vi "LightSheetController_Main.vi"() -> ()   [LabVIEW 2018]
uses:
  VISource/SubVI/ConfigParameters_Analog.ctl
  VISource/SubVI/ConfigParameters_Others1.ctl
  VISource/SubVI/ConfigParameters_Others2.ctl
  VISource/SubVI/ConfigParameters_Digital.ctl
  VISource/SubVI/SetupInfo.ctl
  VISource/SubVI/ProcessParametersOut.ctl
  VISource/SubVI/WaveformParameters.ctl
  VISource/SubVI/AnalogWaveform.ctl
  VISource/SubVI/DigitalWaveform.ctl
  VISource/SubVI/PhysicalResource.ctl
  VISource/SubVI/ControlsRef.ctl
panel:
  in  "FunctionSelect":enum32{"Control Panel", "Settings", "About"}(tab)=enum."Settings"
  in  "XYOnlyMode":bool
  out "RunningMode":string caption="Running Mode"
  in  "QuitRunning":bool
  in  "EXIT":bool
  in  "Mode_1":bool
  in  "Mode_2A":bool
  in  "Mode_2B":bool
  out "ElapsedTime":dbl caption="Elapsed Time" format="%.2f sec"
  in  "EventDetectionMode":bool
  in  "StimulationMode":bool
  out "Messages":string
  in  "ConfigParameters_Digital":T1={"Steps per volume"=25.0, "Time per volume (s)"=0.4, "OG start layer"=23.0, "Objective Lin Rising Vel (micron/ms）"=1.0, "Image depth (micron)"=200.0, "OG latency (s)"=10.0, "OG repitation"=3.0, "OG end layer"=25.0, "Shock1 duration (s)"=0.001, "Shock2 duration (s)"=0.001, "Shock3 duration (s)"=0.01, "Shock4 duration (s)"=0.01, "Shock5 duration (s)"=0.1, "Shock duration_New"=[0.001, 0.001, 0.01, 0.01, 0.1]}
  in  "ConfigParameters_Analog":T2={"JAI camera fps"=100.0, "Bi-Lateral Galvo xy scan range (V)"=0.6, "Bi-Lateral Galvo xy scan frequency (Hz)"=500, "AOM Blind percent (%)"=0.1, "AOM start blind percent (%) "=70.0, "ROI threshold"=3.0, "AO Sampling rate"=500000.0} {"AOM start blind percent (%)" min=10.0 max=90.0; "AOM Blind percent (%)" min=0.1 max=100.0; "Bi-Lateral Galvo xy scan frequency (Hz)" min=500 max=500; "Bi-Lateral Galvo xy scan range (V)" min=0.0 max=1.5}
  in  "ConfigParameters_Other1":T3={"Frontal Galvo xy scan range (V)"=0.14, "Frontal Galvo xy scan frequency (Hz)"=500, "PFI 0 digital clock frequency"=500000.0, "Window size for layer index"=0.5, "sCMOS fps"=95.0} {"Frontal Galvo xy scan frequency (Hz)" min=500 max=500; "Frontal Galvo xy scan range (V)" min=0.0 max=1.5}
  in  "ConfigParameters_Others2":T4={"#Trials baseline"=6, "#Trials test"=6, "Time before acq. (s)"=360.0, "Time before test (s)"=600.0, "#Blocks acquisition"=5, "Inter-trial interval baseline (s)"=60.0, "#Trials per acquition block"=6, "Inter-block interval acquisition (s)"=360.0, "Inter-trial interval acquisition (s)"=20.0, "Flash latency (s)"=20.0, "Flash duration (s)"=3.2, "Response duration (s)"=40.0, "MaxTimeEventDetection (s)"=3600, "StimType"=enum."Flash", "#MaxEvents"=10}
  # "Light Sheet Controller"
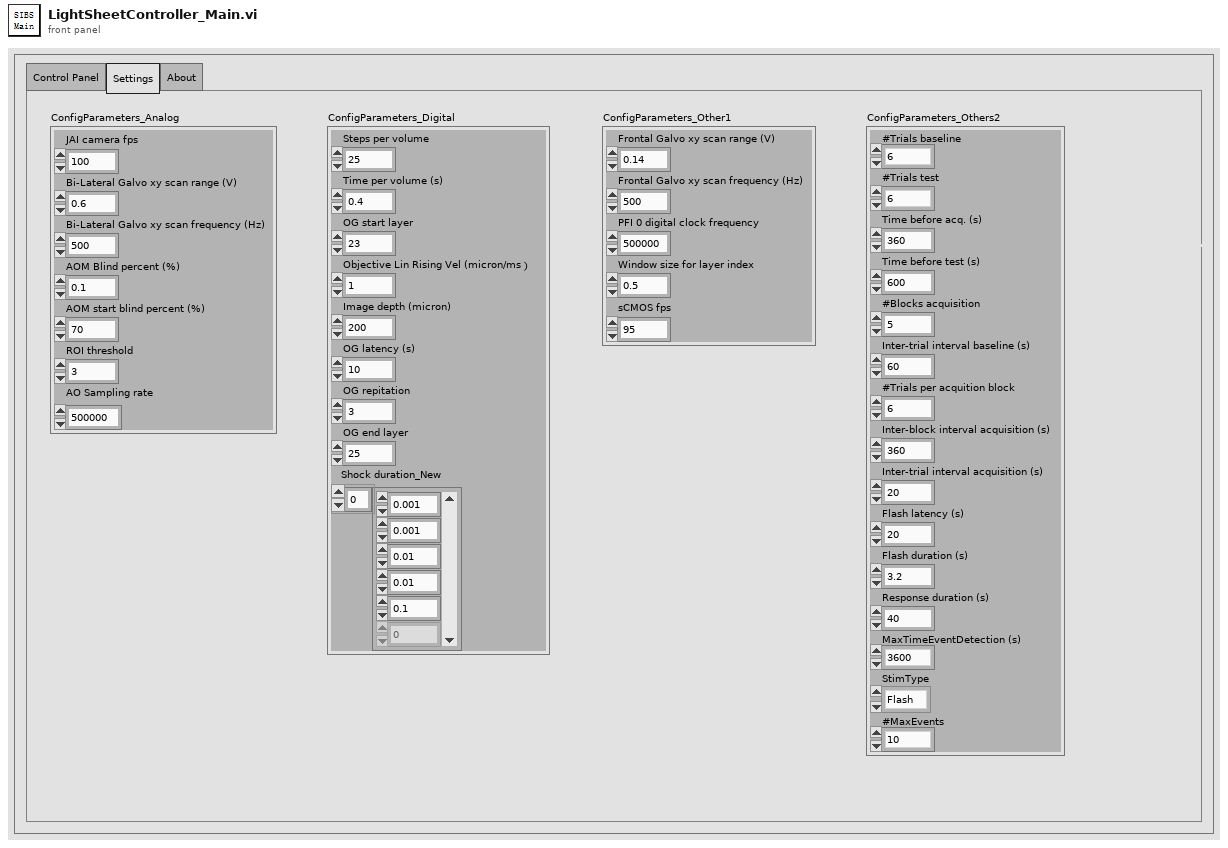
[diagram p1: front panel]
types:
  T1 = typedef "ConfigParameters_Digital.ctl" = cluster{"Steps per volume":dbl, "Time per volume (s)":dbl, "OG start layer":dbl, "Objective Lin Rising Vel (micron/ms）":dbl, "Image depth (micron)":dbl, "OG latency (s)":dbl, "OG repitation":dbl, "OG end layer":dbl, "Shock1 duration (s)":dbl, "Shock2 duration (s)":dbl, "Shock3 duration (s)":dbl, "Shock4 duration (s)":dbl, "Shock5 duration (s)":dbl, "Shock duration_New":dbl[]}
  T2 = typedef "ConfigParameters_Analog.ctl" = cluster{"JAI camera fps":dbl, "Bi-Lateral Galvo xy scan range (V)":dbl, "Bi-Lateral Galvo xy scan frequency (Hz)":i16, "AOM Blind percent (%)":dbl, "AOM start blind percent (%) ":dbl, "ROI threshold":dbl, "AO Sampling rate":dbl}
  T3 = typedef "ConfigParameters_Others1.ctl" = cluster{"Frontal Galvo xy scan range (V)":dbl, "Frontal Galvo xy scan frequency (Hz)":i16, "PFI 0 digital clock frequency":dbl, "Window size for layer index":dbl, "sCMOS fps":dbl}
  T4 = typedef "ConfigParameters_Others2.ctl" = cluster{"#Trials baseline":i32, "#Trials test":i32, "Time before acq. (s)":dbl, "Time before test (s)":dbl, "#Blocks acquisition":i32, "Inter-trial interval baseline (s)":dbl, "#Trials per acquition block":i32, "Inter-block interval acquisition (s)":dbl, "Inter-trial interval acquisition (s)":dbl, "Flash latency (s)":dbl, "Flash duration (s)":dbl, "Response duration (s)":dbl, "MaxTimeEventDetection (s)":i32, "StimType":enum16{"Flash", "OG"}, "#MaxEvents":i32}
  T5 = typedef "SetupInfo.ctl" = cluster{"ConfigParameters_Analog":T2, "ConfigParameters_Digital":T1, "ConfigParameters_Other1":T3, "ConfigParameters_Others2":T4, "ProcessParametersOut":T6, "WaveformParameters":T7, "AnalogWaveform":T8, "DigitalWaveform":T9, "PhysicalResource":T10, "ControlsRef":T11, "test":string}
  T6 = typedef "ProcessParametersOut.ctl" = cluster{"stand Z vol Acquisition time (s)":dbl, "stand Z vol Backward time (s)":dbl, "Objective scan volt":dbl, "Bi-lateral Galvo Z scan volt":dbl, "Frontal Galvo Z scan volt":dbl, "Objective step length (micron)":dbl, "OG Z volet Linear Dec time (s)":dbl, "OG Z vol Stim. steps time (s)":dbl, "OG Z vol Linear Acc time (s)":dbl, "#Vol. of flash":i32, "#Vol. of shock":i32, "#Vol. bef flash":i32, "#Vol. aft flash":i32, "OG Z vol Linear Dec time (s)":dbl, "OG Z vol time (s)":dbl, "Stack duration":dbl[], "AOM stand. value size":i32, "Plane indexing length":i32, "#Vol. blank":i32, "#Vol. blank before acq":i32, "#Vol. blank before test":i32, " #Inter-block interval acquisition (Ed-St Vol)":i32}
  T7 = typedef "WaveformParameters.ctl" = cluster{"stand Z vol Acquisition samp info":cluster{"Fs":dbl, "#s":dbl}, "stand Z vol Backward samp info":cluster{"Fs":dbl, "#s":dbl}, "OG Z vol Linear Acc samp info":cluster{"Fs":dbl, "#s":dbl}, "OG Z vol Stim. steps samp info":cluster{"Fs":dbl, "#s":dbl}, "OG Z volet Linear Dec samp info":cluster{"Fs":dbl, "#s":dbl}, "OG Z vol Linear Dec samp info":cluster{"Fs":dbl, "#s":dbl}, "OG Z vol samp info":cluster{"Fs":dbl, "#s":dbl}, "stand Z vol backforth samp info":cluster{"Fs":dbl, "#s":dbl}}
  T8 = typedef "AnalogWaveform.ctl" = cluster{"Bi-lateral Galvo Z stand waveform":waveform(dbl), "Frontal Galvo Z stand waveform":waveform(dbl), "Bi-lateral Galvo XY stand waveform":waveform(dbl), "Frontal Galvo XY stand waveform":waveform(dbl), "sCMOS stand waveform":waveform(dbl), "Detection objective stand waveform":waveform(dbl), "AOM stand waveform":waveform(dbl), "PFI 0 clock stand waveform":waveform(dbl), "Bi-lateral Galvo Z OG waveform":waveform(dbl), "Bi-lateral Galvo XY OG waveform":waveform(dbl), "Frontal Galvo Z OG waveform":waveform(dbl), "Frontal Galvo XY OG waveform":waveform(dbl), "sCMOS OG waveform":waveform(dbl), "Detection objective OG waveform":waveform(dbl), "AOM OG waveform":waveform(dbl), "PFI 0 clock OG wavee":waveform(dbl), "sCMOS blank waveform":waveform(dbl), "All analog OG wave":waveform(dbl)[], "All analog stand wave":waveform(dbl)[], "All analog blank wave":waveform(dbl)[], "BufferWaveform_Analog":waveform(dbl)[], "Bi-lateral Galvo Z XY":waveform(dbl), "Frontal Galvo Z XY":waveform(dbl), "sCMOS Trigger XY":waveform(dbl), "Detection objective XY":waveform(dbl), "AOM XY":waveform(dbl), "Analog_XY":waveform(dbl)[]}
  T9 = typedef "DigitalWaveform.ctl" = cluster{"AllDigitalStandWave":digitalwaveform[], "AllDigialEvokedWave":digitalwaveform[], "AllDigialOGWave":digitalwaveform[], "AllDigitalPairWave_1":digitalwaveform[], "AllDigitalPairWave_2":digitalwaveform[], "AllDigitalPairWave_3":digitalwaveform[], "AllDigitalPairWave_4":digitalwaveform[], "AllDigitalPairWave_5":digitalwaveform[], "Plane Indexing":digitalwaveform, "Plane indexing P0.5 OG":digitalwaveform, "AllDigitalPairWaves":digitalwaveform[][], "BufferWaveform_Digital":digitalwaveform[], "AllDigitalBlankWave":digitalwaveform[], "Digial_XY":digitalwaveform[], "Digital_XY_flash":digitalwaveform[], "Digial_XY DMD":digitalwaveform[]}
  T10 = typedef "PhysicalResource.ctl" = cluster{"PhysicalChannels_AI":tag, "PhysicalChannels_AO":tag, "PhysicalChannels_DO":tag, "Task_AnalogOutput":refnum<k21>, "Task_DigitalOutput":refnum<k21>, "Task_AnalogInput":refnum<k21>}
  T11 = typedef "ControlsRef.ctl" = cluster{"Mode_1":refnum<vi>, "EventDetectionMode":refnum<vi>, "Mode_2A":refnum<vi>, "StimulationMode":refnum<vi>, "Mode_2B":refnum<vi>, "ErrorMeg":refnum<vi>}
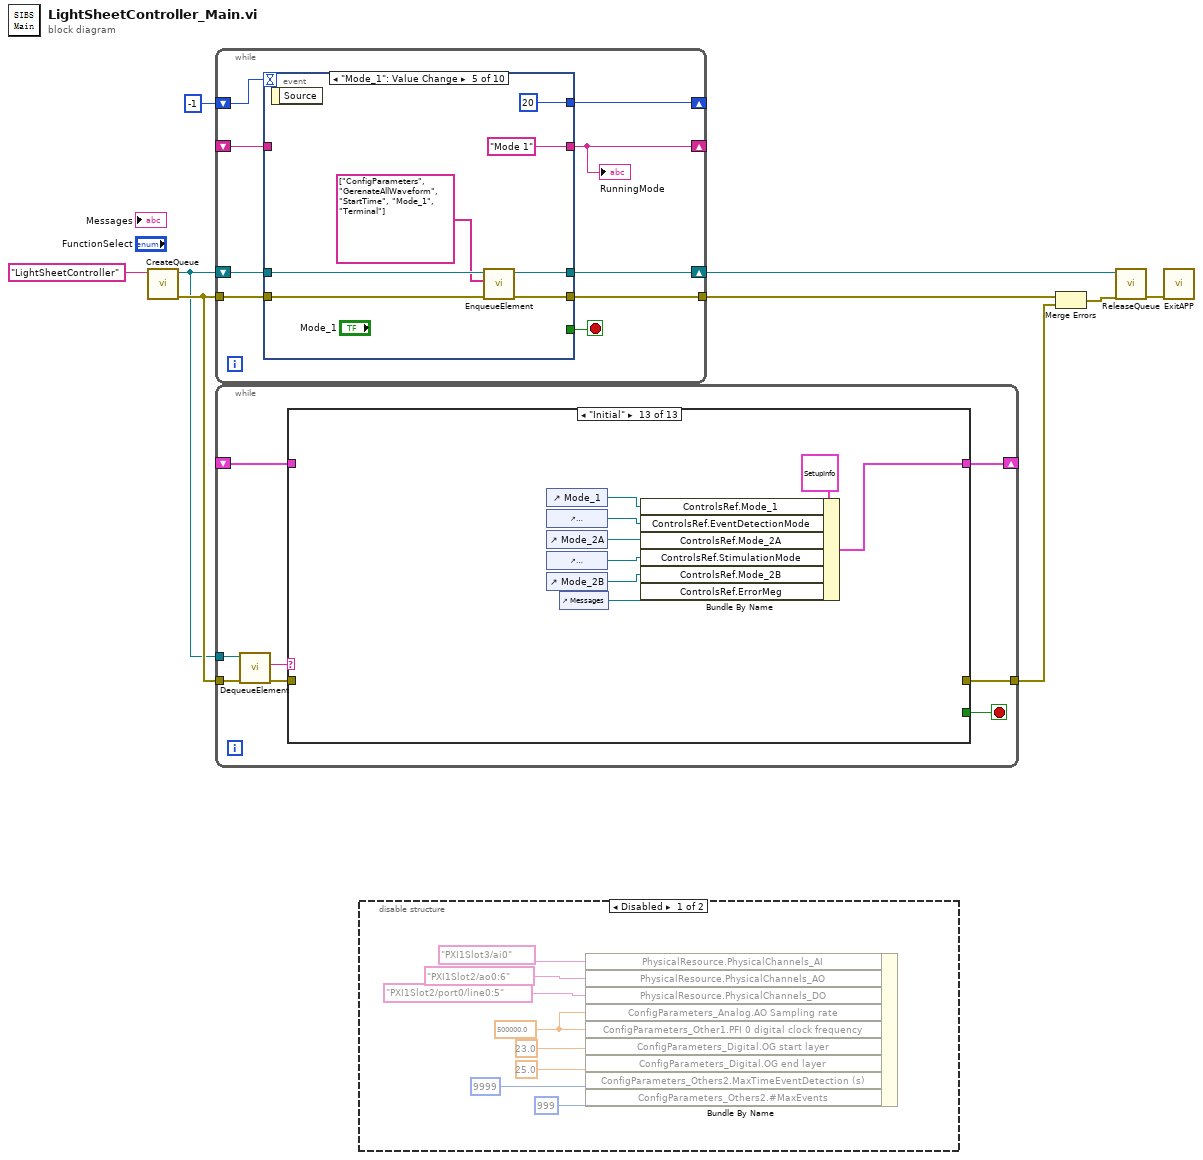
[diagram p0: block diagram]
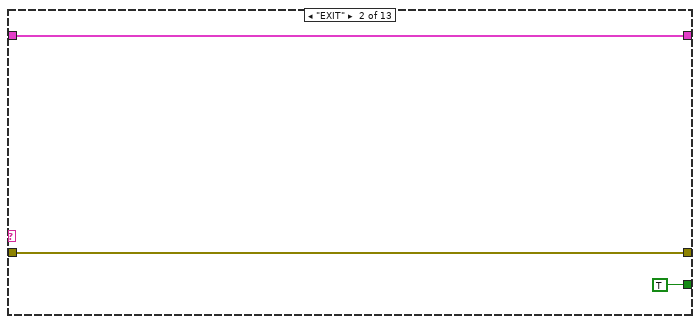
[diagram p4: hidden frame]
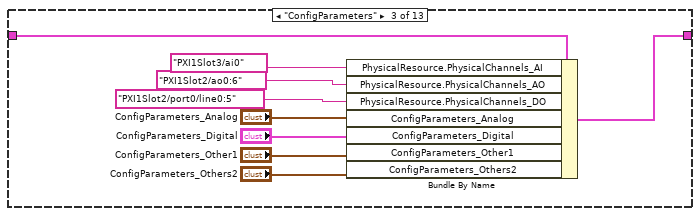
[diagram p5: hidden frame]
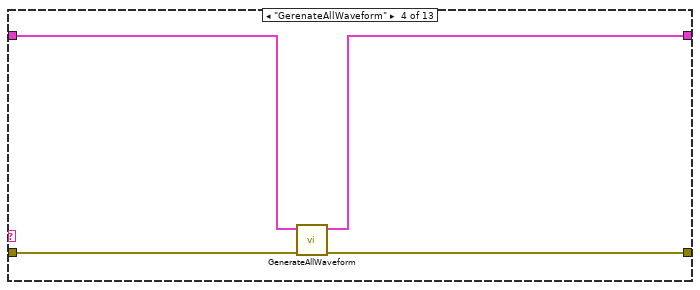
[diagram p6: hidden frame]
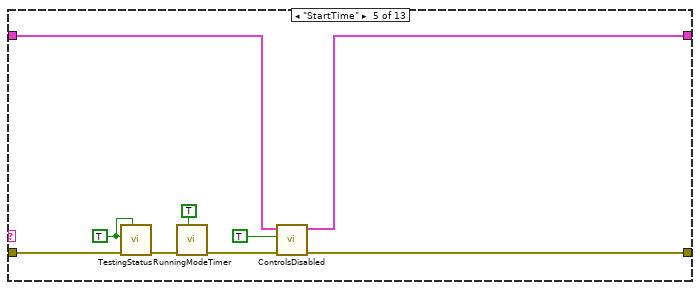
[diagram p7: hidden frame]
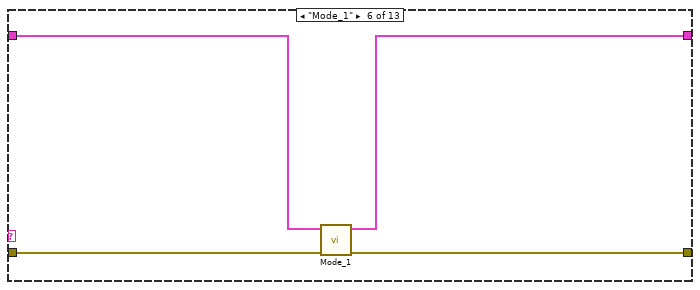
[diagram p8: hidden frame]
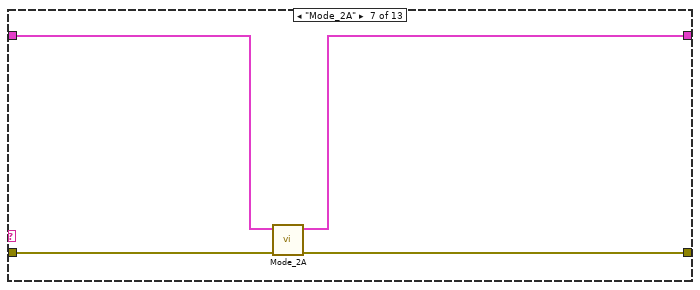
[diagram p9: hidden frame]
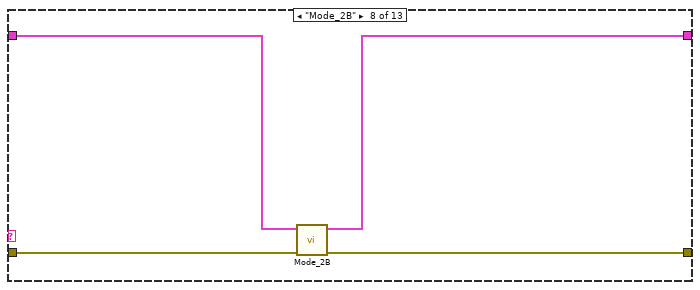
[diagram p10: hidden frame]
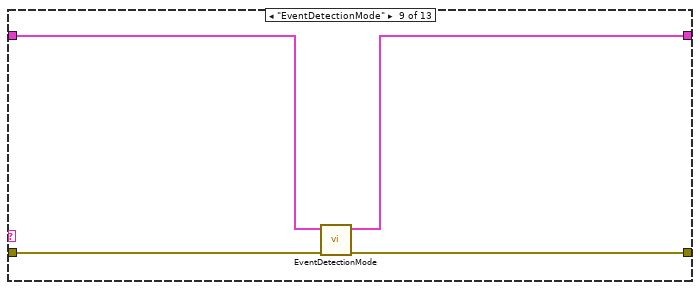
[diagram p11: hidden frame]
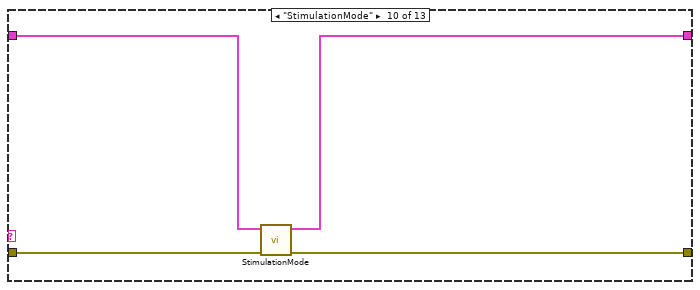
[diagram p12: hidden frame]
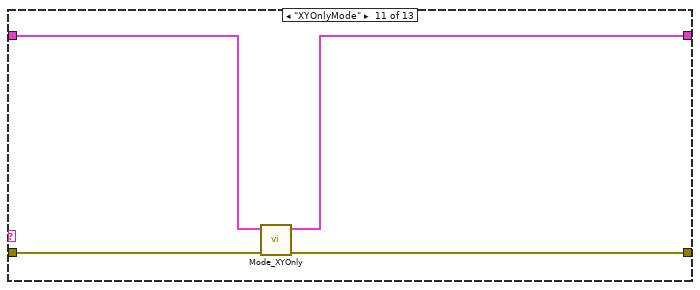
[diagram p13: hidden frame]
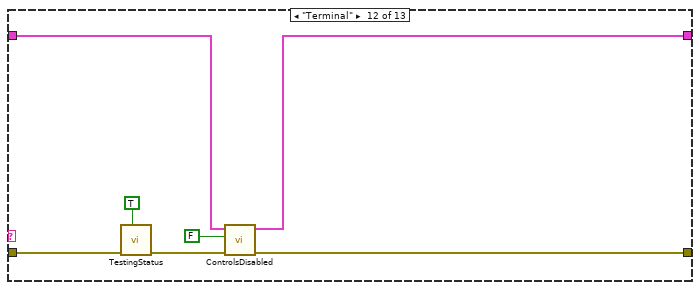
[diagram p14: hidden frame]
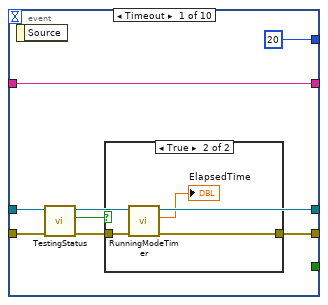
[diagram p15: hidden frame]
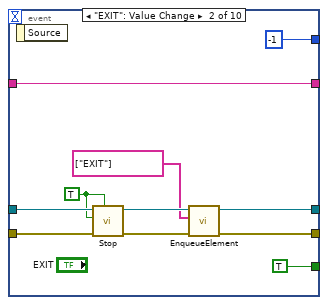
[diagram p17: hidden frame]
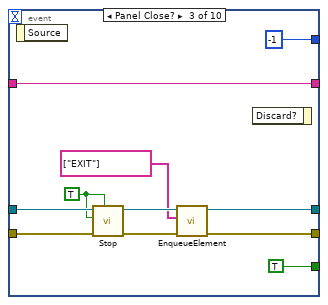
[diagram p18: hidden frame]
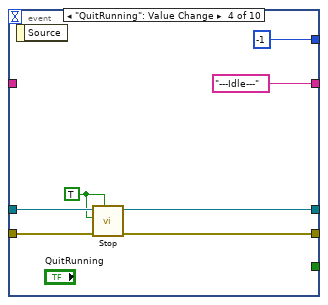
[diagram p19: hidden frame]
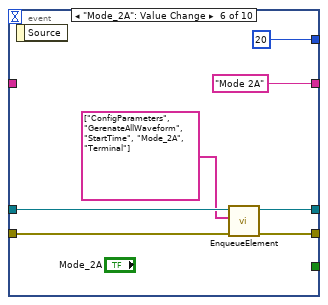
[diagram p20: hidden frame]
diagram:
  n1 = call "CreateQueue.vi"("QueueName"="LightSheetController") -> ("error out"=w9:errorcluster, "QueueOUT"=w8:refnum<queue>)  [unwired: 9 in]
  n2 = while {
    tunnel: w9 -> [w17]
    tunnel: [w16] -> w6
    shift-right: [w14] -> w7
    shift-left: w8 -> [w15]
    shift-right: [w10] -> _
    shift-left: _ -> [w13]
    shift-right: [w11] -> _
    shift-left: -1 -> [w12]
    stop <- w18 stop-if-true
    n3 = event shown="[4] \"Mode_1\": Value Change" {
      selector: _ -> [_ _ _ _ _ _ _ _ _ _]
      dyn-events: _ -> [_ _ _ _ _ _ _ _ _ _]
      timeout: w12 -> [_ _ _ _ _ _ _ _ _ _]
      tunnel: [_ TRUE TRUE _ _ _ _ _ _ _] -> w18
      tunnel: w17 -> [w23 w32 w42 w53 w62 w69 w76 w83 w90 w97]
      tunnel: [w24 w38 w48 w52 w61 w68 w75 w82 w89 w96] -> w16
      tunnel: w15 -> [w25 w37 w47 w55 w60 w67 w74 w81 w88 w95]
      tunnel: [w25 w36 w46 w55 w59 w66 w73 w80 w87 w94] -> w14
      tunnel: [w20 w31 w41 "---Idle---" ("RunningMode") "Mode 1" ("RunningMode") "Mode 2A" ("RunningMode") "Mode 2B" ("RunningMode") "Event Detection Mode" ("RunningMode") "Stimulation Mode" ("RunningMode") "XY Only Mode" ("RunningMode")] -> w10
      tunnel: w13 -> [w20 w31 w41 _ _ _ _ _ _ _]
      tunnel: [20 -1 -1 -1 20 20 20 20 20 20] -> w11
      event Timeout {
        n4 = event-data() -> ()  [unwired: 1 in, 1 out]
        n5 = call "TestingStatus.vi"("error in (no error)"=w23) -> ("error out"=w22:errorcluster, "StateOut"=w21:bool)  [unwired: 9 in]
        n6 = case shown="True" w21 {
          tunnel: [w26 w28] -> w24
          tunnel: w22 -> [w26 w29]
          frame False {
          }
          frame True {
            n7 = call "RunningModeTimer.vi"("error in (no error)"=w29) -> ("error out"=w28:errorcluster, "TimerOut(s)"=→"ElapsedTime":dbl)  [unwired: 9 in]
          }
        }
      }
      event "EXIT": Value Change {
        w34 = TRUE ("Write?")
        n8 = event-data() -> ()  [unwired: 1 in, 1 out]
        n9 = call "Stop.vi"("Write?"=w34, "error in (no error)"=w32, "StateIn"=w34) -> ("error out"=w33:errorcluster)  [unwired: 7 in, 1 out]
        n10 = call "EnqueueElement.vi"("error in (no error)"=w33, "Actions"=string[] ["EXIT"], "QueueIN"=w37) -> ("error out"=w38:errorcluster, "QueueOUT"=w36:refnum<queue>)  [unwired: 7 in]
      }
      event Panel Close? {
        w44 = TRUE ("Write?")
        n11 = event-data() -> ()  [unwired: 1 in, 1 out]
        n12 = call "Stop.vi"("Write?"=w44, "error in (no error)"=w42, "StateIn"=w44) -> ("error out"=w43:errorcluster)  [unwired: 7 in, 1 out]
        n13 = call "EnqueueElement.vi"("error in (no error)"=w43, "Actions"=string[] ["EXIT"], "QueueIN"=w47) -> ("error out"=w48:errorcluster, "QueueOUT"=w46:refnum<queue>)  [unwired: 7 in]
        n14 = event-data() -> ()  [unwired: 2 in, 1 out]
      }
      event "QuitRunning": Value Change {
        w54 = TRUE ("Write?")
        n15 = event-data() -> ()  [unwired: 1 in, 1 out]
        n16 = call "Stop.vi"("Write?"=w54, "error in (no error)"=w53, "StateIn"=w54) -> ("error out"=w52:errorcluster)  [unwired: 7 in, 1 out]
      }
      event "Mode_1": Value Change {
        n17 = event-data() -> ()  [unwired: 1 in, 1 out]
        n18 = call "EnqueueElement.vi"("error in (no error)"=w62, "Actions"=string[] ["ConfigParameters", "GerenateAllWaveform", "StartTime", "Mode_1", "Terminal"], "QueueIN"=w60) -> ("error out"=w61:errorcluster, "QueueOUT"=w59:refnum<queue>)  [unwired: 7 in]
      }
      event "Mode_2A": Value Change {
        n19 = event-data() -> ()  [unwired: 1 in, 1 out]
        n20 = call "EnqueueElement.vi"("error in (no error)"=w69, "Actions"=string[] ["ConfigParameters", "GerenateAllWaveform", "StartTime", "Mode_2A", "Terminal"], "QueueIN"=w67) -> ("error out"=w68:errorcluster, "QueueOUT"=w66:refnum<queue>)  [unwired: 7 in]
      }
      event "Mode_2B": Value Change {
        n21 = event-data() -> ()  [unwired: 1 in, 1 out]
        n22 = call "EnqueueElement.vi"("error in (no error)"=w76, "Actions"=string[] ["ConfigParameters", "GerenateAllWaveform", "StartTime", "Mode_2B", "Terminal"], "QueueIN"=w74) -> ("error out"=w75:errorcluster, "QueueOUT"=w73:refnum<queue>)  [unwired: 7 in]
      }
      event "EventDetectionMode": Value Change {
        n23 = event-data() -> ()  [unwired: 1 in, 1 out]
        n24 = call "EnqueueElement.vi"("error in (no error)"=w83, "Actions"=string[] ["ConfigParameters", "GerenateAllWaveform", "StartTime", "EventDetectionMode", "Terminal"], "QueueIN"=w81) -> ("error out"=w82:errorcluster, "QueueOUT"=w80:refnum<queue>)  [unwired: 7 in]
      }
      event "StimulationMode": Value Change {
        n25 = event-data() -> ()  [unwired: 1 in, 1 out]
        n26 = call "EnqueueElement.vi"("error in (no error)"=w90, "Actions"=string[] ["ConfigParameters", "GerenateAllWaveform", "StartTime", "StimulationMode", "Terminal"], "QueueIN"=w88) -> ("error out"=w89:errorcluster, "QueueOUT"=w87:refnum<queue>)  [unwired: 7 in]
      }
      event "XYOnlyMode": Value Change {
        n27 = event-data() -> ()  [unwired: 1 in, 1 out]
        n28 = call "EnqueueElement.vi"("error in (no error)"=w97, "Actions"=string[] ["ConfigParameters", "GerenateAllWaveform", "StartTime", "XYOnlyMode", "Terminal"], "QueueIN"=w95) -> ("error out"=w96:errorcluster, "QueueOUT"=w94:refnum<queue>)  [unwired: 7 in]
      }
    }
    "RunningMode" <- w10
  }
  n29 = while {
    tunnel: w9 -> [w104]
    tunnel: w8 -> [w103]
    tunnel: [w101] -> w5
    shift-right: [w100] -> _
    shift-left: _ -> [w99]
    stop <- w105 stop-if-true
    n30 = call "DequeueElement.vi"("error in (no error)"=w104, "QueueIN"=w103) -> ("error out"=w102:errorcluster, "Actions"=w98:string)  [unwired: 6 in, 2 out]
    n31 = case shown="\"Initial\"" w98 {
      tunnel: [_ TRUE _ _ _ _ _ _ _ _ _ _ _] -> w105
      tunnel: w102 -> [_ w107 _ w120 w131 w134 w139 w143 w147 w151 w155 w161 _]
      tunnel: [_ w107 _ w119 w126 w132 w136 w141 w145 w148 w152 w158 _] -> w101
      tunnel: [w106 w108 w117 w121 w124 w135 w137 w140 w144 w149 w153 w157 w169] -> w100
      tunnel: w99 -> [w106 w108 w118 w122 w125 w133 w138 w142 w146 w150 w154 w159 _]
      frame "False", Default {
      }
      frame "EXIT" {
      }
      frame "ConfigParameters" {
        n32 = Bundle By Name(cluster=w118, "PhysicalResource.PhysicalChannels_AI"=tag "PXI1Slot3/ai0", "PhysicalResource.PhysicalChannels_AO"=tag "PXI1Slot2/ao0:6", "PhysicalResource.PhysicalChannels_DO"=tag "PXI1Slot2/port0/line0:5", "ConfigParameters_Analog"="ConfigParameters_Analog", "ConfigParameters_Digital"="ConfigParameters_Digital", "ConfigParameters_Other1"="ConfigParameters_Other1", "ConfigParameters_Others2"="ConfigParameters_Others2") -> (w117:T5)
      }
      frame "GerenateAllWaveform" {
        n33 = call "GenerateAllWaveform.vi"("error in (no error)"=w120, "SetupInfo_IN"=w122) -> ("error out"=w119:errorcluster, "SetupInfo_OUT"=w121:T5)  [unwired: 8 in]
      }
      frame "StartTime" {
        w130 = TRUE ("StateIn")
        n34 = call "TestingStatus.vi"("Write?"=w130, "error in (no error)"=w131, "StateIn"=w130) -> ("error out"=w128:errorcluster)  [unwired: 7 in, 1 out]
        n35 = call "RunningModeTimer.vi"("Initial"=TRUE, "error in (no error)"=w128) -> ("error out"=w127:errorcluster)  [unwired: 8 in, 1 out]
        n36 = call "ControlsDisabled.vi"("error in (no error)"=w127, "Disable?"=TRUE, "SetupInfo_IN"=w125) -> ("error out"=w126:errorcluster, "SetupInfo_OUT"=w124:T5)  [unwired: 7 in]
      }
      frame "Mode_1" {
        n37 = call "Mode_1.vi"("error in (no error)"=w134, "SetupInfo_IN"=w133) -> ("error out"=w132:errorcluster, "SetupInfo_OUT"=w135:T5)  [unwired: 8 in]
      }
      frame "Mode_2A" {
        n38 = call "Mode_2A.vi"("error in (no error)"=w139, "SetupInfo_IN"=w138) -> ("error out"=w136:errorcluster, "SetupInfo_OUT"=w137:T5)  [unwired: 8 in]
      }
      frame "Mode_2B" {
        n39 = call "Mode_2B.vi"("error in (no error)"=w143, "SetupInfo_IN"=w142) -> ("error out"=w141:errorcluster, "SetupInfo_OUT"=w140:T5)  [unwired: 8 in]
      }
      frame "EventDetectionMode" {
        n40 = call "EventDetectionMode.vi"("error in (no error)"=w147, "SetupInfo_IN"=w146) -> ("error out"=w145:errorcluster, "SetupInfo_OUT"=w144:T5)  [unwired: 8 in]
      }
      frame "StimulationMode" {
        n41 = call "StimulationMode.vi"("error in (no error)"=w151, "SetupInfo_IN"=w150) -> ("error out"=w148:errorcluster, "SetupInfo_OUT"=w149:T5)  [unwired: 8 in]
      }
      frame "XYOnlyMode" {
        n42 = call "Mode_XYOnly.vi"("error in (no error)"=w155, "SetupInfo_IN"=w154) -> ("error out"=w152:errorcluster, "SetupInfo_OUT"=w153:T5)  [unwired: 8 in]
      }
      frame "Terminal" {
        n43 = call "TestingStatus.vi"("Write?"=TRUE ("StateIn"), "error in (no error)"=w161) -> ("error out"=w160:errorcluster)  [unwired: 8 in, 1 out]
        n44 = call "ControlsDisabled.vi"("error in (no error)"=w160, "Disable?"=FALSE, "SetupInfo_IN"=w159) -> ("error out"=w158:errorcluster, "SetupInfo_OUT"=w157:T5)  [unwired: 7 in]
      }
      frame "Initial" {
        n45 = control-ref of="Mode_1"() -> (w168:refnum<vi>)
        n46 = control-ref of="EventDetectionMode"() -> (w167:refnum<vi>)
        n47 = control-ref of="Mode_2A"() -> (w166:refnum<vi>)
        n48 = control-ref of="StimulationMode"() -> (w165:refnum<vi>)
        n49 = control-ref of="Mode_2B"() -> (w164:refnum<vi>)
        n50 = control-ref of="Messages"() -> (w163:refnum<vi>)
        n51 = Bundle By Name(cluster=T5 {"ConfigParameters_Analog"={"JAI camera fps"=240.0, "Bi-Lateral Galvo xy scan range (V)"=0.7, "Bi-Lateral Galvo xy scan frequency (Hz)"=500, "AOM Blind percent (%)"=0.1, "AOM start blind percent (%) "=70.0, "ROI threshold"=1.0, "AO Sampling rate"=1000000.0}, "ConfigParameters_Digital"={"Steps per volume"=25.0, "Time per volume (s)"=0.4, "OG start layer"=15.0, "Objective Lin Rising Vel (micron/ms）"=1.0, "Image depth (micron)"=200.0, "OG latency (s)"=10.0, "OG repitation"=3.0, "OG end layer"=17.0, "Shock1 duration (s)"=0.001, "Shock2 duration (s)"=0.001, "Shock3 duration (s)"=0.01, "Shock4 duration (s)"=0.01, "Shock5 duration (s)"=0.1, "Shock duration_New"=[0.001, 0.001, 0.01, 0.01, 0.1]}, "ConfigParameters_Other1"={"Frontal Galvo xy scan range (V)"=0.14, "Frontal Galvo xy scan frequency (Hz)"=500, "PFI 0 digital clock frequency"=500000.0, "Window size for layer index"=0.5, "sCMOS fps"=95.0}, "ConfigParameters_Others2"={"#Trials baseline"=6, "#Trials test"=6, "Time before acq. (s)"=360.0, "Time before test (s)"=600.0, "#Blocks acquisition"=5, "Inter-trial interval baseline (s)"=60.0, "#Trials per acquition block"=6, "Inter-block interval acquisition (s)"=360.0, "Inter-trial interval acquisition (s)"=20.0, "Flash latency (s)"=10.0, "Flash duration (s)"=3.2, "Response duration (s)"=10.0, "MaxTimeEventDetection (s)"=6, "StimType"=enum."Flash", "#MaxEvents"=6}, "ProcessParametersOut"={"stand Z vol Acquisition time (s)"=0.2631578947368421, "stand Z vol Backward time (s)"=0.13684210526315793, "Objective scan volt"=5.0, "Bi-lateral Galvo Z scan volt"=0.1800000180000018, "Frontal Galvo Z scan volt"=0.14940000509752818, "Objective step length (micron)"=8.0, "OG Z volet Linear Dec time (s)"=0.024, "OG Z vol Stim. steps time (s)"=0.031578947368421054, "OG Z vol Linear Acc time (s)"=0.112, "#Vol. of flash"=8, "#Vol. of shock"=1, "#Vol. bef flash"=25, "#Vol. aft flash"=17, "OG Z vol Linear Dec time (s)"=0.112, "OG Z vol time (s)"=0.39073684210526316, "Stack duration"=[0.001, 0.001, 0.01, 0.01, 0.1], "AOM stand. value size"=400000, "Plane indexing length"=0, "#Vol. blank"=0, "#Vol. blank before acq"=1000000, "#Vol. blank before test"=263158, " #Inter-block interval acquisition (Ed-St Vol)"=1000000}, "WaveformParameters"={"stand Z vol Acquisition samp info"={"Fs"=1000000.0, "#s"=263158.0}, "stand Z vol Backward samp info"={"Fs"=1000000.0, "#s"=136842.0}, "OG Z vol Linear Acc samp info"={"Fs"=1000000.0, "#s"=112000.0}, "OG Z vol Stim. steps samp info"={"Fs"=1000000.0, "#s"=31579.0}, "OG Z volet Linear Dec samp info"={"Fs"=1000000.0, "#s"=24000.0}, "OG Z vol Linear Dec samp info"={"Fs"=1000000.0, "#s"=112000.0}, "OG Z vol samp info"={"Fs"=1000000.0, "#s"=390737.0}, "stand Z vol backforth samp info"={"Fs"=1000000.0, "#s"=400000.0}}, "AnalogWaveform"={"Bi-lateral Galvo Z stand waveform"={"t0"=timestamp(0 s since 1904-01-01), "dt"=1.0, "Y"=[]}, "Frontal Galvo Z stand waveform"={"t0"=timestamp(0 s since 1904-01-01), "dt"=1.0, "Y"=[]}, "Bi-lateral Galvo XY stand waveform"={"t0"=timestamp(0 s since 1904-01-01), "dt"=1.0, "Y"=[]}, "Frontal Galvo XY stand waveform"={"t0"=timestamp(0 s since 1904-01-01), "dt"=1.0, "Y"=[]}, "sCMOS stand waveform"={"t0"=timestamp(0 s since 1904-01-01), "dt"=1.0, "Y"=[]}, "Detection objective stand waveform"={"t0"=timestamp(0 s since 1904-01-01), "dt"=1.0, "Y"=[]}, "AOM stand waveform"={"t0"=timestamp(0 s since 1904-01-01), "dt"=1.0, "Y"=[]}, "PFI 0 clock stand waveform"={"t0"=timestamp(0 s since 1904-01-01), "dt"=1.0, "Y"=[]}, "Bi-lateral Galvo Z OG waveform"={"t0"=timestamp(0 s since 1904-01-01), "dt"=1.0, "Y"=[]}, "Bi-lateral Galvo XY OG waveform"={"t0"=timestamp(0 s since 1904-01-01), "dt"=1.0, "Y"=[]}, "Frontal Galvo Z OG waveform"={"t0"=timestamp(0 s since 1904-01-01), "dt"=1.0, "Y"=[]}, "Frontal Galvo XY OG waveform"={"t0"=timestamp(0 s since 1904-01-01), "dt"=1.0, "Y"=[]}, "sCMOS OG waveform"={"t0"=timestamp(0 s since 1904-01-01), "dt"=1.0, "Y"=[]}, "Detection objective OG waveform"={"t0"=timestamp(0 s since 1904-01-01), "dt"=1.0, "Y"=[]}, "AOM OG waveform"={"t0"=timestamp(0 s since 1904-01-01), "dt"=1.0, "Y"=[]}, "PFI 0 clock OG wavee"={"t0"=timestamp(0 s since 1904-01-01), "dt"=1.0, "Y"=[]}, "sCMOS blank waveform"={"t0"=timestamp(0 s since 1904-01-01), "dt"=1.0, "Y"=[]}, "All analog OG wave"=[], "All analog stand wave"=[], "All analog blank wave"=[], "BufferWaveform_Analog"=[], "Bi-lateral Galvo Z XY"={"t0"=timestamp(0 s since 1904-01-01), "dt"=1.0, "Y"=[]}, "Frontal Galvo Z XY"={"t0"=timestamp(0 s since 1904-01-01), "dt"=1.0, "Y"=[]}, "sCMOS Trigger XY"={"t0"=timestamp(0 s since 1904-01-01), "dt"=1.0, "Y"=[]}, "Detection objective XY"={"t0"=timestamp(0 s since 1904-01-01), "dt"=1.0, "Y"=[]}, "AOM XY"={"t0"=timestamp(0 s since 1904-01-01), "dt"=1.0, "Y"=[]}, "Analog_XY"=[]}, "DigitalWaveform"={"AllDigitalStandWave"=[], "AllDigialEvokedWave"=[], "AllDigialOGWave"=[], "AllDigitalPairWave_1"=[], "AllDigitalPairWave_2"=[], "AllDigitalPairWave_3"=[], "AllDigitalPairWave_4"=[], "AllDigitalPairWave_5"=[], "Plane Indexing"={"t0"=timestamp(0 s since 1904-01-01), "dt"=0.0, "Y"={"transitions"=[], "data"=[]}, "error"={"status"=FALSE, "code"=37421928, "source"=""}}, "Plane indexing P0.5 OG"={"t0"=timestamp(0 s since 1904-01-01), "dt"=0.0, "Y"={"transitions"=[], "data"=[]}, "error"={"status"=FALSE, "code"=37421928, "source"=""}}, "AllDigitalPairWaves"=[], "BufferWaveform_Digital"=[], "AllDigitalBlankWave"=[], "Digial_XY"=[], "Digital_XY_flash"=[], "Digial_XY DMD"=[]}, "PhysicalResource"={"PhysicalChannels_AI"="", "PhysicalChannels_AO"="", "PhysicalChannels_DO"="", "Task_AnalogOutput"="", "Task_DigitalOutput"="", "Task_AnalogInput"=""}, "ControlsRef"={"Mode_1"=refnum, "EventDetectionMode"=refnum, "Mode_2A"=refnum, "StimulationMode"=refnum, "Mode_2B"=refnum, "ErrorMeg"=refnum}, "test"=""} ("SetupInfo_IN"), "ControlsRef.Mode_1"=w168, "ControlsRef.EventDetectionMode"=w167, "ControlsRef.Mode_2A"=w166, "ControlsRef.StimulationMode"=w165, "ControlsRef.Mode_2B"=w164, "ControlsRef.ErrorMeg"=w163) -> (w169:T5)
      }
    }
  }
  n52 = disable-structure shown="Disabled" {
    frame Disabled {
      w174 = 500000.0 ("ConfigParameters_Analog.AO Sampling rate")
      n53 = Bundle By Name("PhysicalResource.PhysicalChannels_AI"=tag "PXI1Slot3/ai0", "PhysicalResource.PhysicalChannels_AO"=tag "PXI1Slot2/ao0:6", "PhysicalResource.PhysicalChannels_DO"=tag "PXI1Slot2/port0/line0:5", "ConfigParameters_Analog.AO Sampling rate"=w174, "ConfigParameters_Other1.PFI 0 digital clock frequency"=w174, "ConfigParameters_Digital.OG start layer"=23.0, "ConfigParameters_Digital.OG end layer"=25.0, "ConfigParameters_Others2.MaxTimeEventDetection (s)"=9999, "ConfigParameters_Others2.#MaxEvents"=999) -> ()  [unwired: 1 in, 1 out]
    }
    frame Enabled {
    }
  }
  n54 = Merge Errors(w6, w5) -> (w4:errorcluster)
  n55 = call "ReleaseQueue.vi"("error in (no error)"=w4, "QueueIN"=w7) -> ("error out"=w2:errorcluster)  [unwired: 9 in]
  n56 = call "ExitAPP.vi"("error in (no error)"=w2) -> ()  [unwired: 10 in, 1 out]
